vi "FRCts20_WebMethods_Notifications_POST.vi"(7 "LabVIEW Web Service Request":refnum<class "Web Request.lvclass">) -> ()   [LabVIEW 2014, in "FRCts20_WebMethods.lvlib"]
uses:
  FRCts20_WebMethods.lvlib
  <vilib>/wsapi/Web Request.lvclass
  Backend/source/VI Source/FRCts20_Backend_API/SNS.ctl
  Backend/source/VI Source/FRCts20_Backend_API/ApiReturn.ctl
  Backend/source/VI Source/FRCts20_Backend_API/FRCts20_Backend_API_SNS.ctl
  Backend/source/VI Source/FRCts20_Backend_API/FRCts20_Backend_API_Command_SNS.ctl
  Backend/source/VI Source/FRCts20_Backend_API/FRCts20_Backend_API_SNS.vi
  Backend/source/VI Source/FRCts20_Backend_API/FRCts20_Backend_API.lvlib
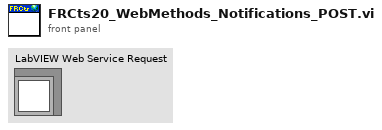
[diagram p1: front panel]
types:
  T1 = typedef "FRCts20_Backend_Engine.lvlib/FRCts20_Backend_API.lvlib/SNS.ctl" = cluster{"APIReturn":T2, "SNS":T3}
  T2 = typedef "FRCts20_Backend_Engine.lvlib/FRCts20_Backend_API.lvlib/ApiReturn.ctl" = string
  T3 = typedef "FRCts20_Backend_Engine.lvlib/FRCts20_Backend_API.lvlib/FRCts20_Backend_API_SNS.ctl" = cluster{"EventIndexes":i32[], "TeamNumber":u32, "Subject":string, "MainMessage":string, "Phone#":string, "Email":string, "Request Index":i32}
  T4 = typedef "FRCts20_Backend_Engine.lvlib/FRCts20_Backend_API.lvlib/FRCts20_Backend_API_Command_SNS.ctl" = string
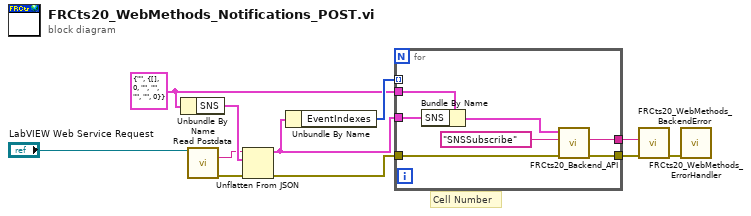
[diagram p0: block diagram]
diagram:
  w1 = T1 {"APIReturn"="", "SNS"={"EventIndexes"=[], "TeamNumber"=0, "Subject"="", "MainMessage"="", "Phone#"="", "Email"="", "Request Index"=0}} ("Event In")
  # "Cell Number"
  n1 = Unbundle By Name(w1) -> ("SNS"=w6:T3)
  n2 = call <vilib>:"Read Postdata.vi"("LabVIEW Web Service Request"="LabVIEW Web Service Request") -> ("postdata"=w5:string, "error out"=w8:errorcluster)  [unwired: 12 in, 1 out]
  n3 = Unflatten From JSON(JSON string=w5, type and defaults=w6, error in (no error)=w8) -> (value=w3:T3, error out=w7:errorcluster)  [unwired: 4 in]
  n4 = Unbundle By Name(w3) -> ("EventIndexes"=w4:i32[])
  n5 = for {
    tunnel: w7 -> [w18]
    tunnel: [w17] -> w11
    tunnel: [w16] -> w10
    tunnel: w4 -> [_] mode=indexing
    tunnel: w3 -> [w13]
    tunnel: w1 -> [w12]
    n6 = Bundle By Name(cluster=w12, "SNS"=w13) -> (w14:T1)
    n7 = call-poly "FRCts20_Backend_API.vi"("error in (no error)"=w18, "SNS"=T4 "SNSSubscribe", "SNS In"=w14) -> ("error out"=w17:errorcluster, "Status"=w16:string)  [unwired: 6 in, 1 out]
  }
  n8 = call "FRCts20_WebMethods_BackendError.vi"("error in (no error)"=w11, "Status"=w10) -> ("error out"=w2:errorcluster)  [unwired: 8 in, 1 out]
  n9 = call "FRCts20_WebMethods_ErrorHandler.vi"("error in"=w2) -> ()  [unwired: 9 in, 2 out]
